vi "Vision Research Phantom Series PhCon PhSetPartitions.vi"(0 "CN in":u32=1, 1 "Count":u32=1, 3 "pWeights":u32[](array[numeric]), 5 "Error In (no error)":errorcluster) -> (14 "CN out":u32=1, 19 "Error Out":errorcluster)   [LabVIEW 2013, in "VRI.lvlib"]
doc: "PhCon.dll\n\nPhSetPartitions\nHRESULT PhSetPartitions(UINT CN, UINT Count, PUINT pWeights);\n\nParameters Description\nCN (in) Camera number.\nCount (in) Count of partitions.\npWeights (in) Array of weights of the memory size to be allocated to each cine.\n To get the percent of each partition multiply its weight by 100 \n and divide by the sum of all weights.\nReturn HRESULT (0=Ok)\nComments Define partitions of the camera memory for multicine recording (v7).\n All recorded cines are deleted when this function is called.\n\nWritten by:\nBLOOMY CONTROLS, INC\nWINDSOR, CT 06095, USA\n860-298-9925\nwww.bloomy.com\nV1.0.0\nMay, 2004"
uses:
  VRI.lvlib
  Phantom DLLs/PhCon.dll
panel:
  # "For instructions on the use of this VI, press Ctrl+H to display the help window and move the mouse over the icon, controls, and indicators"
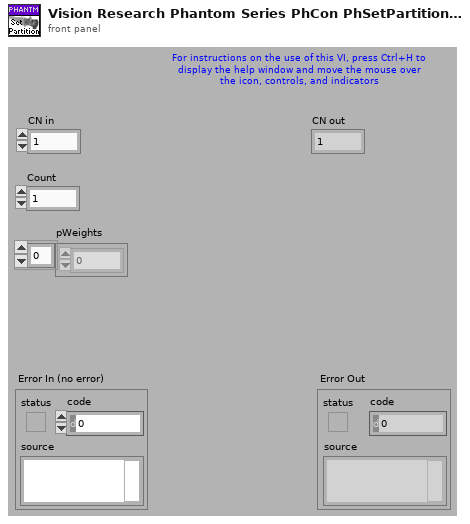
[diagram p1: front panel]
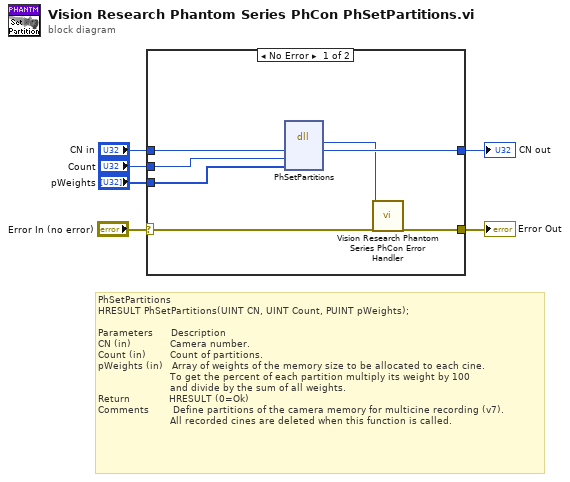
[diagram p0: block diagram]
diagram:
  # "PhSetPartitions\nHRESULT PhSetPartitions(UINT CN, UINT Count, PUINT pWeights);\n\nParameters      Description\nCN (in)             Camera number.\nCount (in)        Count of partitions.\npWeights (in)   Array of weights of the memory size to be allocated to each cine.\n                        To get the percent of each partition multiply its weight by 100 \n                        and divide by the sum of all weights.\nReturn             HRESULT (0=Ok)\nComments        Define partitions of the camera memory for multicine recording (v7).\n                        All recorded cines are deleted when this function is called."
  n1 = case shown="No Error" "Error In (no error)" {
    selector: "Error In (no error)" -> [w13 w15]
    tunnel: [w12 w15] -> w5
    tunnel: "CN in" -> [w11 w14]
    tunnel: [w10 w14] -> w3
    tunnel: "Count" -> [w9 _]
    tunnel: "pWeights" -> [w8 _]
    frame No Error {
      n2 = dll-call lib="C:/Projects/SDK/32-bit/Vision Research Phantom Series Labview Driver/Phantom DLLs/PhCon.dll" fn="PhSetPartitions"("CN"=w11, "Count"=w9, "pWeights"=w8) -> ("HRESULT"=w7:i32, "CN"=w10:u32)  [unwired: 5 in, 2 out]
      n3 = call "Vision Research Phantom Series PhCon Error Handler.vi"("ErrNo"=w7, "Error In (no error)"=w13) -> ("Error Out"=w12:errorcluster)  [unwired: 17 out]
    }
    frame Error {
    }
  }
  "Error Out" <- w5
  "CN out" <- w3
